vi "MultiRows to one row.vi"(8 "error in (no error)":errorcluster, 11 "MultRow String":string) -> (0 "error out":errorcluster, 1 "Array":string[](array[string]), 2 "Final size(s)":i32, 3 "One Row String":string)   [LabVIEW 2021]
panel:
  out "Original array":string[](array[string])
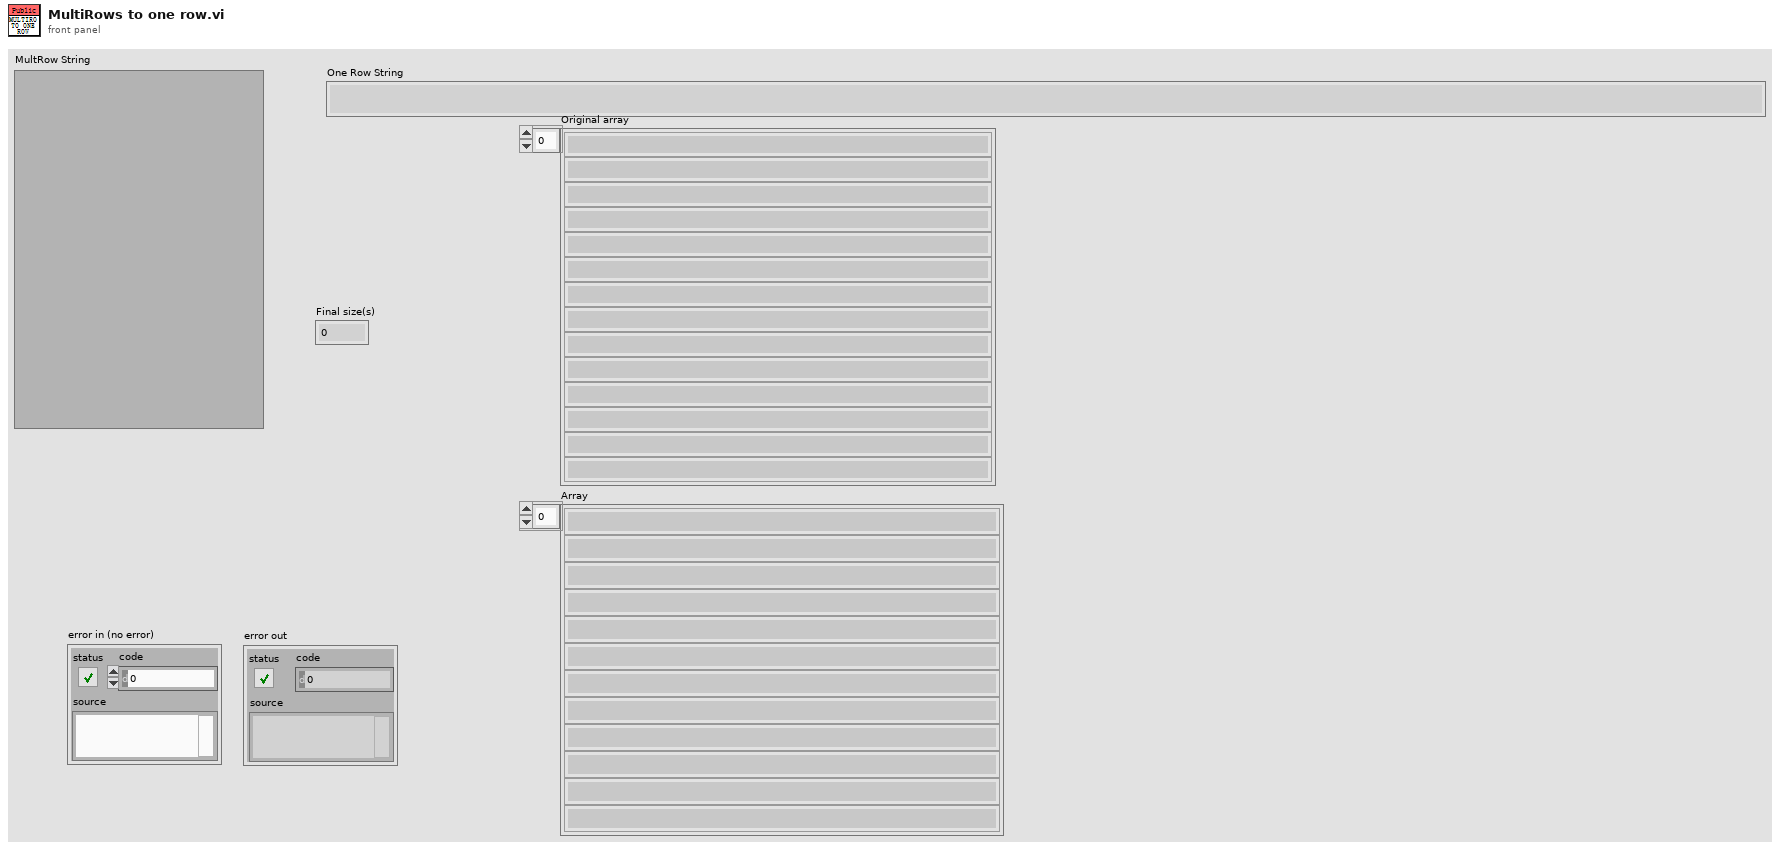
[diagram p1: front panel]
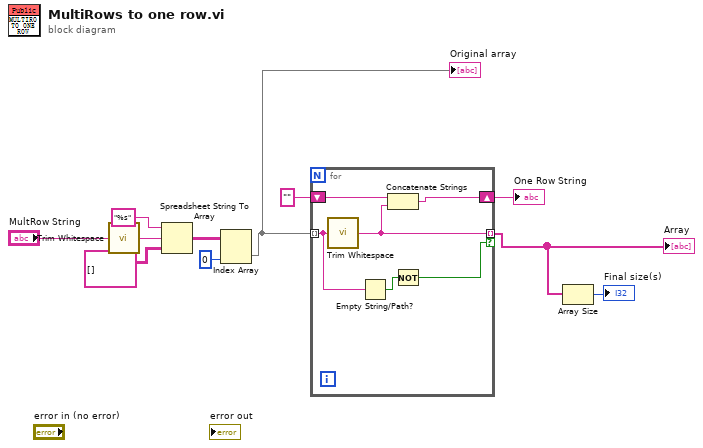
[diagram p0: block diagram]
diagram:
  n1 = call <vilib>:"Trim Whitespace.vi"("string"="MultRow String") -> ("trimmed string"=w5:string)  [unwired: 1 in]
  n2 = Spreadsheet String To Array(format string="%s", spreadsheet string=w5, array type (2D Dbl)=string[][] []) -> (array=w7:string[][])  [unwired: 1 in]
  n3 = Index Array(array=w7, index (col)=0 ("disabled index (col)")) -> (element=w3:string[])  [unwired: 1 in]
  "Original array" <- w3
  n4 = for {
    tunnel: w3 -> [w15] mode=indexing
    shift-right: [w16] -> w11
    shift-left: "" -> [w17]
    tunnel: [w14] -> w1 mode=indexing if=w12
    n5 = call <vilib>:"Trim Whitespace.vi"("string"=w15) -> ("trimmed string"=w14:string)  [unwired: 1 in]
    n6 = Empty String/Path?(string/path=w15) -> (empty?=w13:bool)
    n7 = Concatenate Strings(w17, w14) -> (w16:string)
    n8 = Not(x=w13) -> (.not. x?=w12:bool)
  }
  "One Row String" <- w11
  "Array" <- w1
  n9 = Array Size(array=w1) -> (size(s)=→"Final size(s)":i32)
